vi "Write Error Log.vi"(6 "Log File Path":string, 7 "Site Number":i32, 8 "error in":errorcluster, 9 "Details":string, 10 "Location Message":string, 11 "Code Message":string) -> (0 "error out":errorcluster, 3 "Error Log Path":path)   [LabVIEW 2014, in "TSM Runtime Error Logger.lvlib"]
uses:
  TSM Runtime Error Logger.lvlib
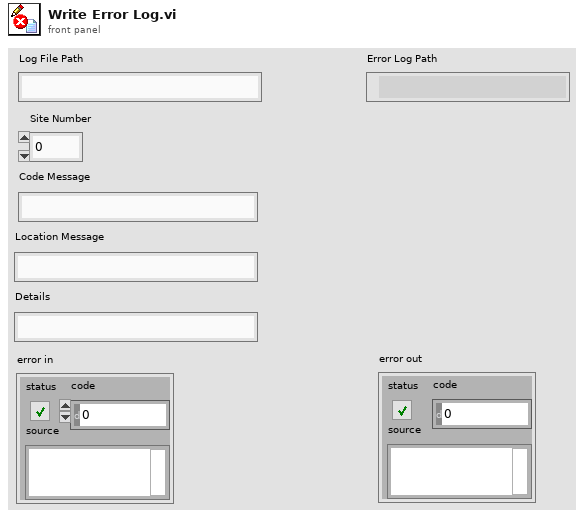
[diagram p1: front panel]
types:
  T1 = enum16{"open", "replace", "create", "open or create", "replace or create", "replace or create with confirmation"}
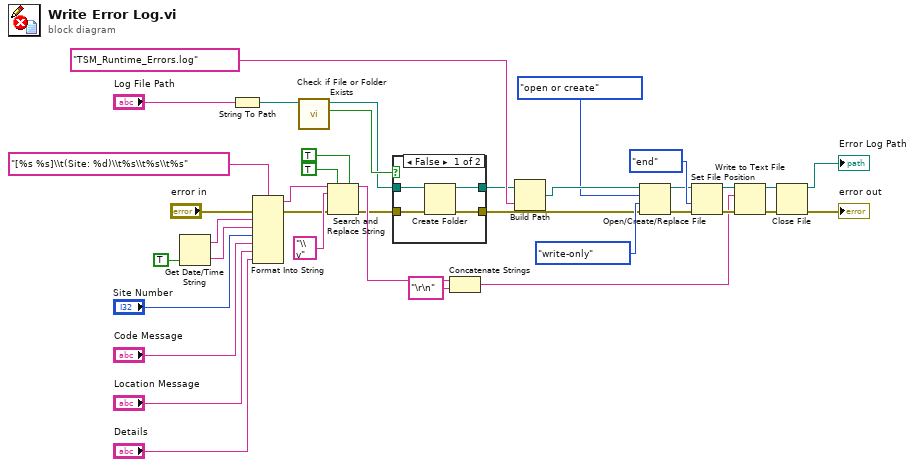
[diagram p0: block diagram]
diagram:
  n1 = Get Date/Time String(want seconds? (F)=TRUE) -> (date string=w35:string, time string=w34:string)  [unwired: 2 in]
  n2 = String To Path(string="Log File Path") -> (path=w2:path)
  n3 = Format Into String(format string="[%s %s]\\t(Site: %d)\\t%s\\t%s\\t%s", error in="error in", w35, w34, "Site Number", "Code Message", "Location Message", "Details") -> (resulting string=w15:string, error out=w12:errorcluster)  [unwired: 1 in]
  n4 = call <vilib>:"Check if File or Folder Exists.vi"("path"=w2) -> ("file or folder exists?"=w8:bool, "dup path"=w5:path)  [unwired: 8 in, 1 out]
  n5 = Search and Replace String(replace all?=TRUE ("replace all? (F)"), multiline?=TRUE ("ignore case? (F)"), input string=w15, search string="\\v" ("string"), error in=w12) -> (result string=w13:string, error out=w7:errorcluster)  [unwired: 3 in, 2 out]
  n6 = case shown="False" w8 {
    tunnel: w7 -> [w41 w42]
    tunnel: [w40 w42] -> w6
    tunnel: w5 -> [w39 w43]
    tunnel: [w38 w43] -> w4
    frame False {
      n7 = Create Folder(path (use dialog)=w39, error in=w41) -> (created path=w38:path, error out=w40:errorcluster)  [unwired: 1 in, 1 out]
    }
    frame True {
    }
  }
  n8 = Concatenate Strings(w13, "\r\n" ("string")) -> (w17:string)
  n9 = Build Path(base path=w4, name or relative path="TSM_Runtime_Errors.log") -> (appended path=w20:path)
  n10 = Open/Create/Replace File(file path (use dialog)=w20, error in=w6, operation (0:open)=T1."open or create", access (0:read/write)=enum16{"read/write", "read-only", "write-only"}."write-only") -> (refnum out=w23:refnum<file>, error out=w25:errorcluster)  [unwired: 2 in, 1 out]
  n11 = Set File Position(refnum=w23, from (0:start)=enum16{"start", "end", "current"}."end", error in=w25) -> (refnum out=w22:refnum<file>, error out=w24:errorcluster)  [unwired: 1 in]
  n12 = Write to Text File(file (use dialog)=w22, text=w17, error in=w24) -> (refnum out=w27:refnum<file>, error out=w28:errorcluster)  [unwired: 1 in, 1 out]
  n13 = Close File(refnum=w27, error in=w28) -> (path=→"Error Log Path":path, error out=→"error out":errorcluster)
